vi "set control settings.vi"(8 "error in (no error)":errorcluster, 10 "control_settings":T1, 11 "id":i32) -> (0 "error out":errorcluster, 3 "function return":i32)   [LabVIEW 2012, in "libximc.lvlib"]
doc: "result_t XIMC_API set_control_settings (device_t id, const control_settings_t* control_settings);"
uses:
  libximc.lvlib
  libximc.dll
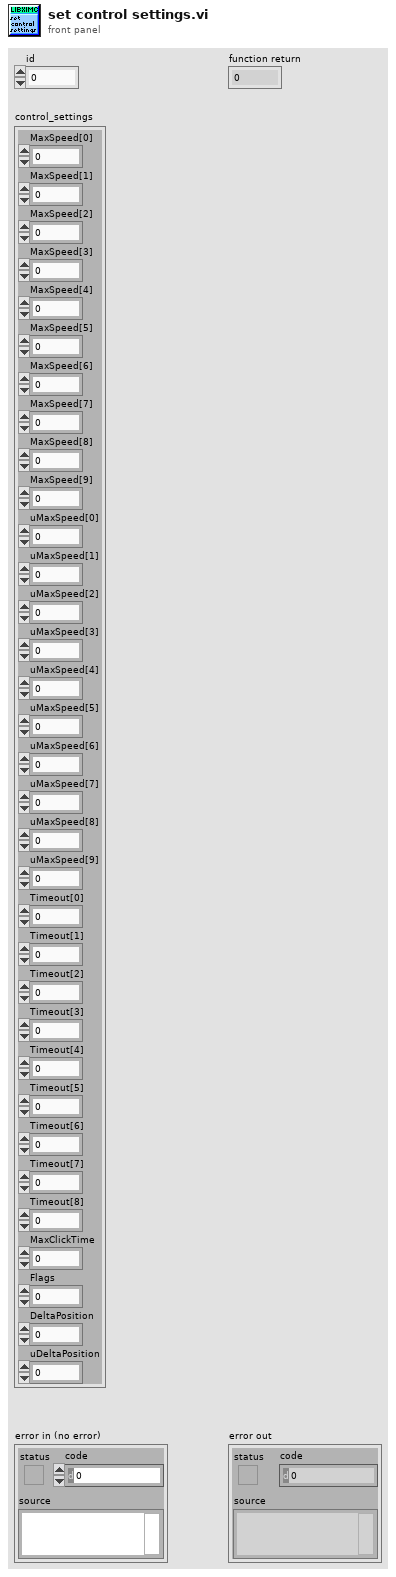
[diagram p1: front panel]
types:
  T1 = cluster{"MaxSpeed[0]":u32, "MaxSpeed[1]":u32, "MaxSpeed[2]":u32, "MaxSpeed[3]":u32, "MaxSpeed[4]":u32, "MaxSpeed[5]":u32, "MaxSpeed[6]":u32, "MaxSpeed[7]":u32, "MaxSpeed[8]":u32, "MaxSpeed[9]":u32, "uMaxSpeed[0]":u32, "uMaxSpeed[1]":u32, "uMaxSpeed[2]":u32, "uMaxSpeed[3]":u32, "uMaxSpeed[4]":u32, "uMaxSpeed[5]":u32, "uMaxSpeed[6]":u32, "uMaxSpeed[7]":u32, "uMaxSpeed[8]":u32, "uMaxSpeed[9]":u32, "Timeout[0]":u32, "Timeout[1]":u32, "Timeout[2]":u32, "Timeout[3]":u32, "Timeout[4]":u32, "Timeout[5]":u32, "Timeout[6]":u32, "Timeout[7]":u32, "Timeout[8]":u32, "MaxClickTime":u32, "Flags":u32, "DeltaPosition":i32, "uDeltaPosition":i32}
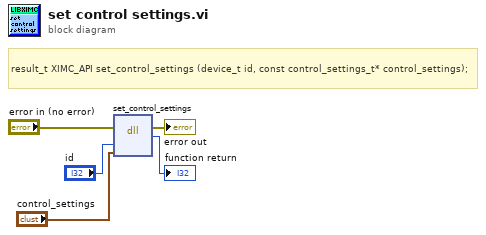
[diagram p0: block diagram]
diagram:
  # "result_t XIMC_API set_control_settings (device_t id, const control_settings_t* control_settings);"
  n1 = dll-call lib="C:/Users/user/Desktop/labview-2.9.11-gen/libximc.*" fn="set_control_settings"(error in="error in (no error)", "id"="id", "control_settings"="control_settings") -> (error out=→"error out":errorcluster, →"function return":i32)  [unwired: 4 in, 1 out]
